vi "Sliding_Mean.vi"(0 "[IN] Buffer":dbl[](array[numeric]), 1 "[IN] Iteration / # Measurment":i32, 2 "[IN] Current Measure":dbl) -> (5 "[OUT] Sliding Average":dbl)   [LabVIEW 2022 SP3]
uses:
  <vilib>/Analysis/NI_AALBase.lvlib
  <vilib>/Analysis/baseanly.llb/Mean (DBL).vi
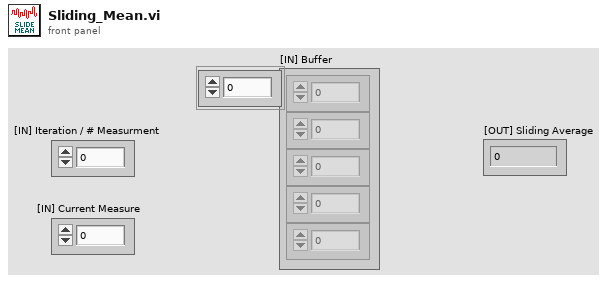
[diagram p1: front panel]
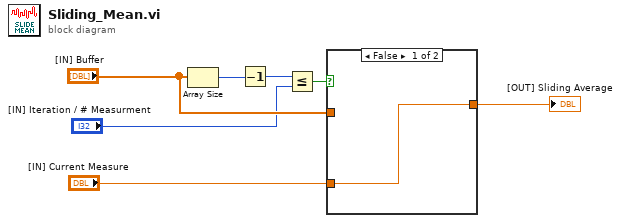
[diagram p0: block diagram]
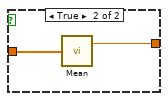
[diagram p2: hidden frame]
diagram:
  n1 = Array Size(array="[IN] Buffer") -> (size(s)=w7:i32)
  n2 = Decrement(x=w7) -> (x-1=w4:i32)
  n3 = Less Or Equal?(x=w4, y="[IN] Iteration / # Measurment") -> (x <= y?=w2:bool)
  n4 = case shown="False" w2 {
    tunnel: "[IN] Current Measure" -> [w8 _]
    tunnel: "[IN] Buffer" -> [_ w10]
    tunnel: [w8 w9] -> w1
    frame False {
    }
    frame True {
      n5 = call-poly <vilib>:"Mean.vi"("X"=w10) -> ("mean"=w9:dbl)  [unwired: 1 out]
    }
  }
  "[OUT] Sliding Average" <- w1
